vi "Close Oscilloscope.vi"(8 "error in (no error)":errorcluster, 11 "Tektonix 2000 in":refnum<class "Tektonix 2000.lvclass">) -> (0 "error out":errorcluster, 3 "Tektonix 2000 out 2":refnum<class "Tektonix 2000.lvclass">)   [LabVIEW 2020, in "Osciloscope Tektronix.lvlib" / "Tektonix 2000.lvclass"]
uses:
  Tektonix 2000.lvclass
  C:/Users/Pablo/Osciloscope-Tek/TDS2000/Libraries/Osciloscope Tektronix/Clases/Osciloscope/Osciloscope.lvclass
  Osciloscope/Osciloscope.lvclass/Osciloscope.ctl
  Osciloscope/Read COM.vi
  <instrlib>/Tektronix TDS 200 1000 2000 Series/Tektronix TDS 200 1000 2000 Series.lvlib
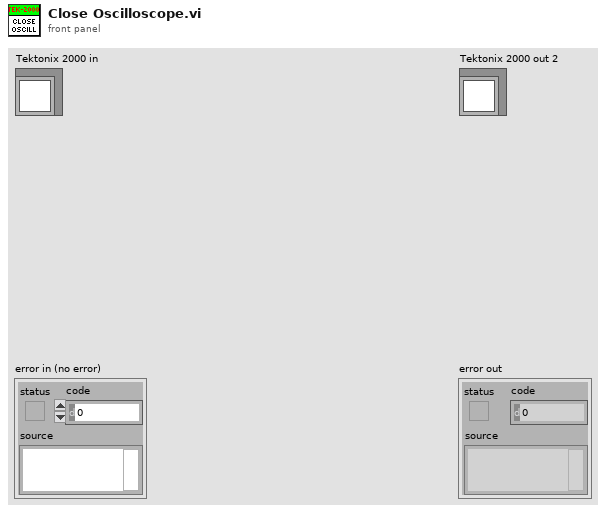
[diagram p1: front panel]
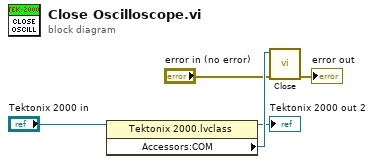
[diagram p0: block diagram]
diagram:
  n1 = property class="Tektonix 2000.lvclass"(reference="Tektonix 2000 in") -> (reference out=→"Tektonix 2000 out 2":refnum<class "Tektonix 2000.lvclass">, "Accessors:COM"=w4:refnum<visa-resource-name>)  [unwired: 1 in, 1 out]
  n2 = call <instrlib>:"Close.vi"("error in (no error)"="error in (no error)", "VISA resource name"=w4) -> ("error out"=→"error out":errorcluster)  [unwired: 9 in]
